vi "generate unique file or folder name.vi"(8 "error in":errorcluster, 11 "file/folder path in":path) -> (0 "error out":errorcluster, 3 "path out":path)   [LabVIEW 2020, in "Reusable Library.lvlib"]
doc: "Returns unique file or folder path which does not existes in system.\nUsed for preventing overwriting of files and folders\n\nBy Samuel James"
uses:
  Reusable Library.lvlib
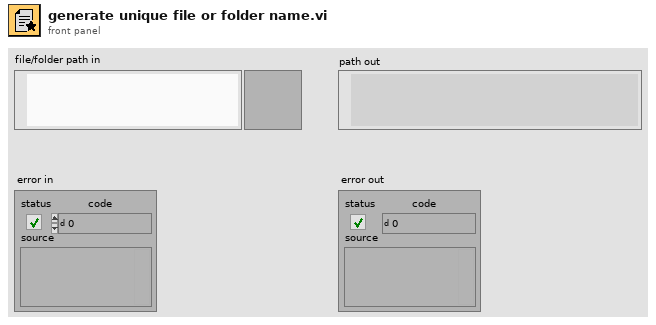
[diagram p1: front panel]
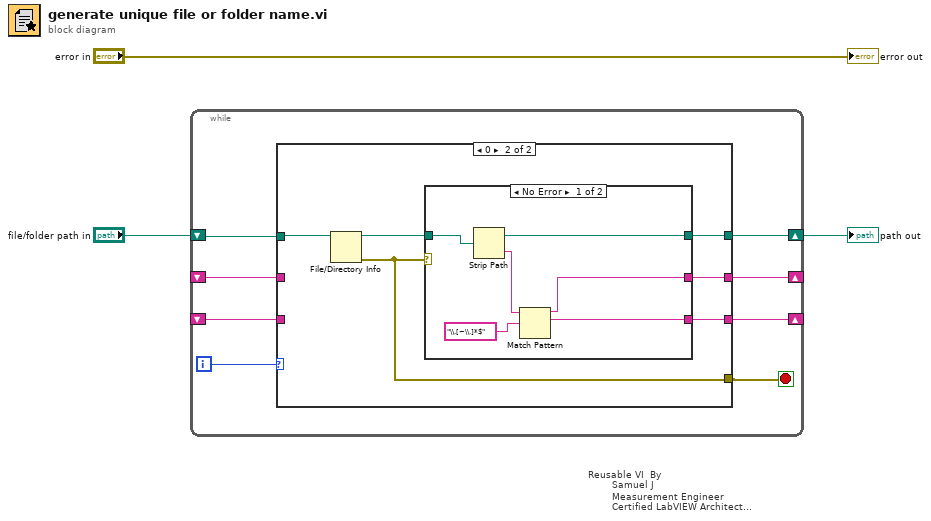
[diagram p0: block diagram]
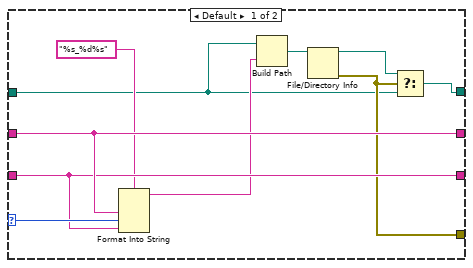
[diagram p2: hidden frame]
diagram:
  n1 = while "Reusable VI  By\n        Samuel J\n        Measurement Engineer\n        Certified LabVIEW Architect\n        Vestas Technology R&D Chennai" {
    shift-right: [w9] -> w2
    shift-left: "file/folder path in" -> [w10]
    shift-right: [w8] -> _
    shift-left: _ -> [w6]
    shift-right: [w7] -> _
    shift-left: _ -> [w5]
    i -> [w11]
    stop <- w4 stop-if-true
    n2 = case shown="0" w11 {
      selector: w11 -> [w20 _]
      tunnel: w10 -> [w13 w27]
      tunnel: [w12 w26] -> w9
      tunnel: [w21 w24] -> w8
      tunnel: [w19 w23] -> w7
      tunnel: w6 -> [w21 _]
      tunnel: w5 -> [w19 _]
      tunnel: [w15 w22] -> w4
      frame Default {
        n3 = Format Into String(format string="%s_%d%s", w21, w20, w19) -> (resulting string=w18:string)  [unwired: 2 in, 1 out]
        n4 = Build Path(base path=w13, name or relative path=w18) -> (appended path=w16:path)
        n5 = File/Directory Info(path=w16) -> (path out=w14:path, error out=w15:errorcluster)  [unwired: 1 in, 5 out]
        n6 = Select(t=w14, s=w15, f=w13) -> (s? t:f=w12:path)
      }
      frame 0 {
        n7 = File/Directory Info(path=w27) -> (path out=w25:path, error out=w22:errorcluster)  [unwired: 1 in, 5 out]
        n8 = case shown="No Error" w22 {
          tunnel: [w32 w34] -> w26
          tunnel: w25 -> [w33 w34]
          tunnel: [w29 _] -> w24
          tunnel: [w28 _] -> w23
          frame No Error {
            n9 = Strip Path(path=w33) -> (stripped path=w32:path, name=w31:string)
            n10 = Match Pattern(string=w31, regular expression="\\.[~\\.]*$") -> (before substring=w29:string, match substring=w28:string)  [unwired: 3 out]
          }
          frame Error {
          }
        }
      }
    }
  }
  "path out" <- w2
  "error out" <- "error in"
